vi "Custom_Create_VI_Icon_Image.vi"(8 "error in (no error)":errorcluster, 9 "Image Depth":i32=24, 10 "Image Format (jpeg)":enum32{"PNG", "JPEG", "GIF"}(ring)=enum."JPEG", 11 "VI":refnum<vi>) -> (0 "error out":errorcluster, 3 "Path to image":path)   [LabVIEW 2019]
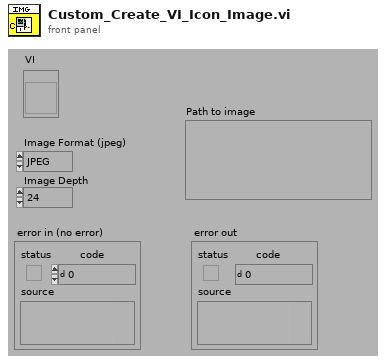
[diagram p1: front panel]
types:
  T1 = cluster{"Printing:Custom All Controls?":bool, "Printing:Custom Connector?":bool, "Printing:Custom Control Descriptions?":bool, "Printing:Custom Control Types?":bool, "Printing:Custom Controls?":bool, "Printing:Custom Description?":bool, "Printing:Custom Diagram Hidden?":bool, "Printing:Custom Diagram Repeat?":bool, "Printing:Custom Diagram?":bool, "Printing:Custom Hierarchy?":bool, "Printing:Custom History?":bool, "Printing:Custom Panel Border?":bool, "Printing:Custom Panel?":bool, "Printing:Custom SubVIs?":bool}
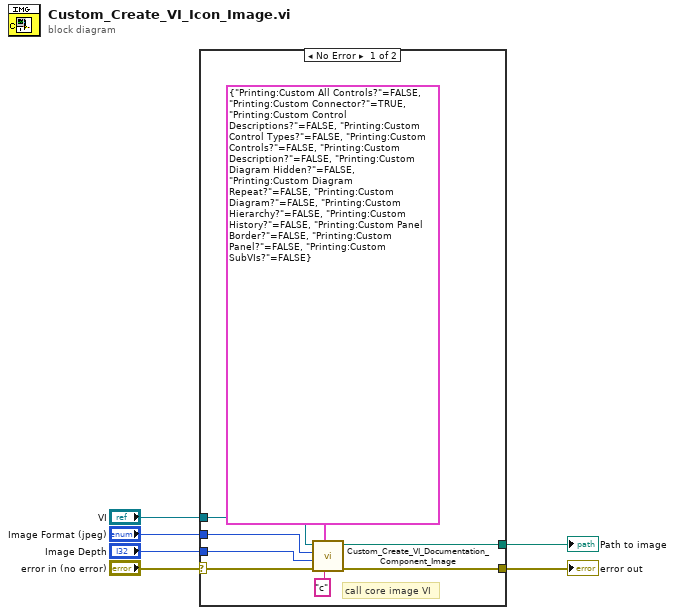
[diagram p0: block diagram]
diagram:
  n1 = case shown="No Error" "error in (no error)" {
    selector: "error in (no error)" -> [w7 w15]
    tunnel: "VI" -> [w14 _]
    tunnel: "Image Format (jpeg)" -> [w13 _]
    tunnel: "Image Depth" -> [w12 _]
    tunnel: [w11 _] -> w3
    tunnel: [w10 w15] -> w2
    frame No Error {
      # "call core image VI"
      n2 = call "Custom_Create_VI_Documentation_Component_Image.vi"("special chars in file path of image"="c", "Content Options"=T1 {"Printing:Custom All Controls?"=FALSE, "Printing:Custom Connector?"=TRUE, "Printing:Custom Control Descriptions?"=FALSE, "Printing:Custom Control Types?"=FALSE, "Printing:Custom Controls?"=FALSE, "Printing:Custom Description?"=FALSE, "Printing:Custom Diagram Hidden?"=FALSE, "Printing:Custom Diagram Repeat?"=FALSE, "Printing:Custom Diagram?"=FALSE, "Printing:Custom Hierarchy?"=FALSE, "Printing:Custom History?"=FALSE, "Printing:Custom Panel Border?"=FALSE, "Printing:Custom Panel?"=FALSE, "Printing:Custom SubVIs?"=FALSE}, "error in (no error)"=w7, "Image Depth"=w12, "Image Format (jpeg)"=w13, "VI"=w14) -> ("error out"=w10:errorcluster, "Path to image"=w11:path)  [unwired: 4 in]
    }
    frame Error {
    }
  }
  "error out" <- w2
  "Path to image" <- w3
